vi "ReadCom.vi"(8 "error in (no error)":errorcluster, 10 "delay before read (ms)":u32=500, 11 "Com In":refnum<visa-resource-name>) -> (0 "error out":errorcluster, 1 "Response":string, 2 "bytes read":u32, 3 "Com Out":refnum<visa-resource-name>)   [LabVIEW 2014]
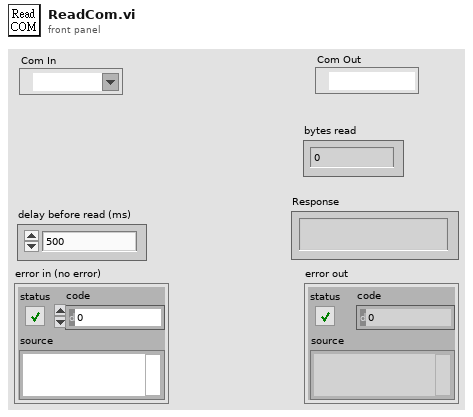
[diagram p1: front panel]
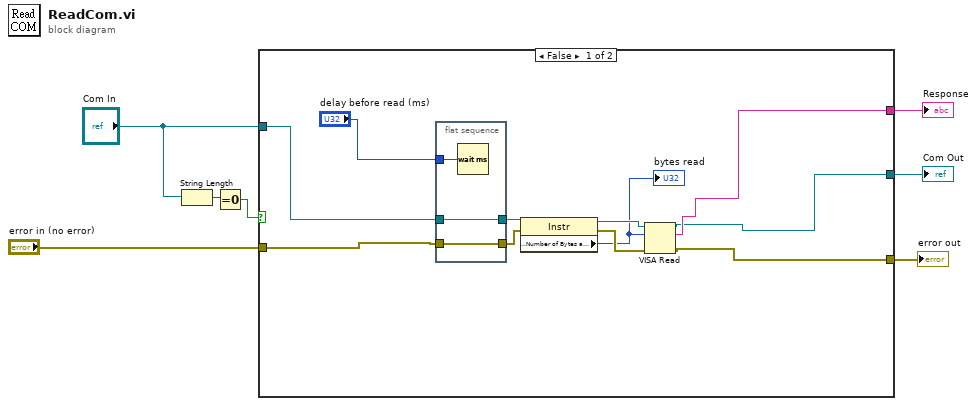
[diagram p0: block diagram]
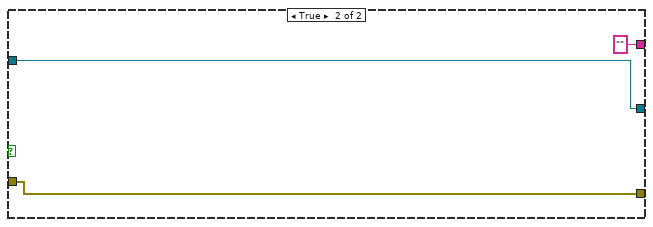
[diagram p2: hidden frame]
diagram:
  n1 = String Length(string="Com In") -> (length=w2:i32)
  n2 = Equal To 0?(x=w2) -> (x = 0?=w1:bool)
  n3 = case shown="False" w1 {
    tunnel: "error in (no error)" -> [w17 w22]
    tunnel: "Com In" -> [w15 w23]
    tunnel: [w10 "" ("read buffer")] -> w6
    tunnel: [w9 w23] -> w5
    tunnel: [w8 w22] -> w4
    frame False {
      n4 = flat-sequence {
        tunnel: w17 -> [w20]
        tunnel: [w20] -> w16
        tunnel: w15 -> [w19]
        tunnel: [w19] -> w14
        tunnel: "delay before read (ms)" -> [w21]
        frame #0 {
          n5 = Wait (ms)(milliseconds to wait=w21) -> ()  [unwired: 1 out]
        }
      }
      n6 = property class="Instr"(reference=w14, error in=w16) -> (reference out=w13:refnum<visa-resource-name>, error out=w12:errorcluster, "Serial Settings:Number of Bytes at Serial Port"=w11:u32)
      "bytes read" <- w11
      n7 = VISA Read(VISA resource name=w13, byte count=w11, error in (no error)=w12) -> (VISA resource name out=w9:refnum<visa-resource-name>, read buffer=w10:string, error out=w8:errorcluster)  [unwired: 1 out]
    }
    frame True {
    }
  }
  "error out" <- w4
  "Response" <- w6
  "Com Out" <- w5
